vi "Wait on Connection.vi"(8 "error in (no error)":errorcluster, 9 "timeout (ms)":i32=200, 11 "TCP_Streamer in":refnum<class "TCP_Streamer_Publisher.lvclass">=refnum) -> (0 "error out":errorcluster, 3 "TCP_Streamer out":refnum<class "TCP_Streamer_Publisher.lvclass">)   [LabVIEW 2021, in "TCP_Streamer_Publisher.lvclass"]
uses:
  TCP_Streamer_Publisher.lvclass
  TCP_Streamer_Publisher.lvclass/TCP_Streamer_Publisher.ctl
  Typedef/State.ctl
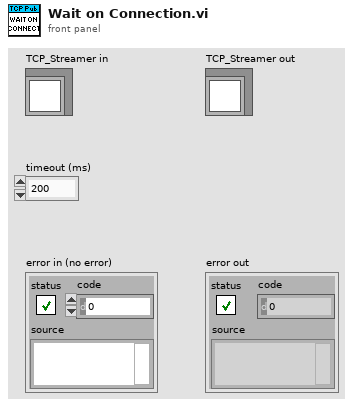
[diagram p1: front panel]
types:
  T1 = typedef "TCP_Streamer_Publisher.lvclass/State.ctl" = enum16{"Stopped", "Listening", "Ready for Data", "Ready to Send", "Sending"}
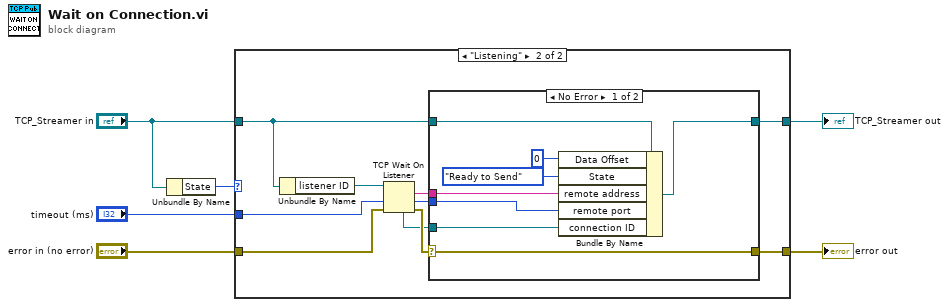
[diagram p0: block diagram]
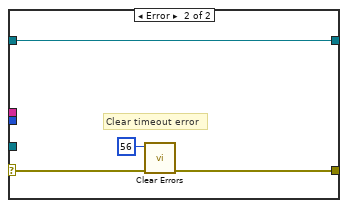
[diagram p3: hidden frame]
diagram:
  n1 = Unbundle By Name("TCP_Streamer in") -> ("State"=w6:T1)
  n2 = case shown="\"Listening\"" w6 {
    tunnel: "TCP_Streamer in" -> [w8 w14]
    tunnel: [w8 w10] -> w4
    tunnel: "timeout (ms)" -> [_ w17]
    tunnel: "error in (no error)" -> [w7 w16]
    tunnel: [w7 w9] -> w1
    frame "Stopped", Default {
    }
    frame "Listening" {
      n3 = Unbundle By Name(w14) -> ("listener ID"=w18:refnum<k5>)
      n4 = TCP Wait On Listener(8:w16, 9:w17, 11:w18) -> (0:w15:errorcluster, 1:w11:u16, 2:w13:string, 4:w12:refnum<k5>)  [unwired: 1 in, 1 out]
      n5 = case shown="No Error" w15 {
        selector: w15 -> [w20 w29]
        tunnel: w14 -> [w26 w30]
        tunnel: w13 -> [w25 _]
        tunnel: w12 -> [w23 _]
        tunnel: w11 -> [w24 _]
        tunnel: [w21 w30] -> w10
        tunnel: [w20 w28] -> w9
        frame No Error {
          n6 = Bundle By Name(cluster=w26, "Data Offset"=0, "State"=State."Ready to Send", "remote address"=w25, "remote port"=w24, "connection ID"=w23) -> (w21:refnum<class "TCP_Streamer_Publisher.lvclass">)
        }
        frame Error {
          # "Clear timeout error"
          n7 = call <vilib>:"Clear Errors.vi"("error in (no error)"=w29, "specific error code to clear (0: all)"=56) -> ("error out"=w28:errorcluster)  [unwired: 4 in, 1 out]
        }
      }
    }
  }
  "error out" <- w1
  "TCP_Streamer out" <- w4
